vi "SetUSB5DoImmediately.vi"(8 "错误输入（无错误）":errorcluster, 9 "Value":u32, 10 "Chan":u32=1, 11 "DevIndex":i32) -> (0 "错误输出":errorcluster, 3 "DevIndex Out":i32)   [LabVIEW 2020]
uses:
  lib/x64/USB5000.dll
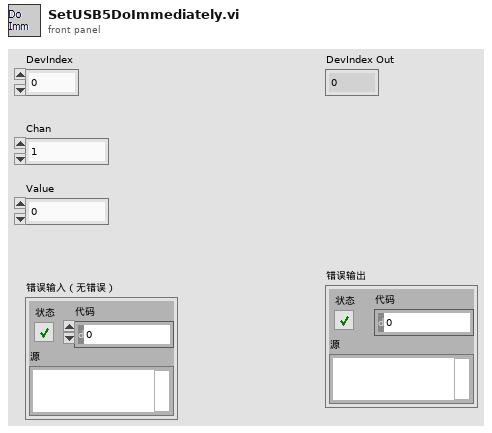
[diagram p1: front panel]
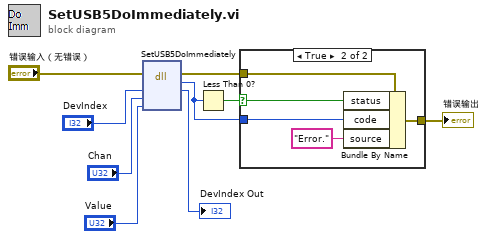
[diagram p0: block diagram]
diagram:
  n1 = dll-call lib="C:/Users/phosense/Downloads/USB-5000/USB-5000_LabVIEW/lib/x64/USB5000.dll" fn="SetUSB5DoImmediately"(error in="错误输入（无错误）", "DevIndex"="DevIndex", "Chan"="Chan", "Value"="Value") -> (error out=w4:errorcluster, "返回类型"=w3:i32, "DevIndex"=→"DevIndex Out":i32)  [unwired: 4 in, 1 out]
  n2 = Less Than 0?(x=w3) -> (x < 0?=w5:bool)
  n3 = case shown="True" w5 {
    selector: w5 -> [_ w11]
    tunnel: [w10 w13] -> w2
    tunnel: w3 -> [_ w15]
    tunnel: w4 -> [w10 w12]
    frame False {
    }
    frame True {
      n4 = Bundle By Name(cluster=w12, "status"=w11, "code"=w15, "source"="Error." ("error message (\"\")")) -> (w13:errorcluster)
    }
  }
  "错误输出" <- w2
